vi "Radau5_Sim Time Check.vi"(8 "error in (no error)":errorcluster, 9 "Allow reverse?":bool, 10 "Final time":dbl, 11 "Initial time":dbl) -> (0 "error out":errorcluster)   [LabVIEW 2017, in "NI_DAE.lvlib"]
uses:
  <vilib>/gmath/NI_DAE.lvlib
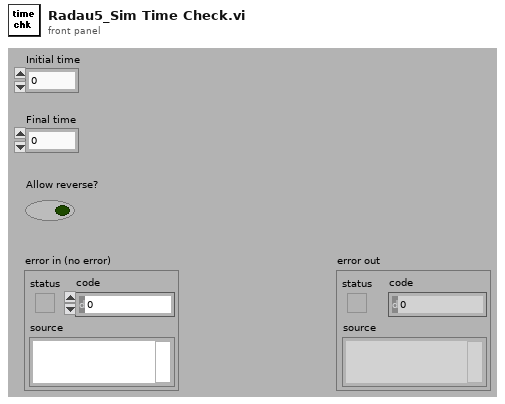
[diagram p1: front panel]
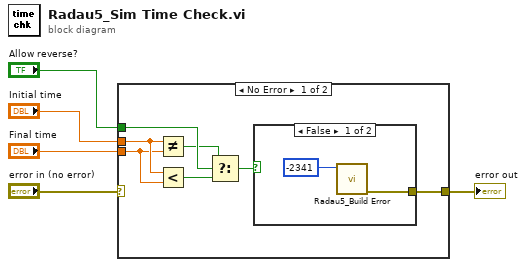
[diagram p0: block diagram]
diagram:
  n1 = case shown="No Error" "error in (no error)" {
    selector: "error in (no error)" -> [_ w15]
    tunnel: "Initial time" -> [w12 _]
    tunnel: "Final time" -> [w11 _]
    tunnel: "Allow reverse?" -> [w10 _]
    tunnel: [w6 w15] -> w1
    frame No Error {
      n2 = Not Equal?(x=w12, y=w11) -> (x != y?=w9:bool)
      n3 = Less?(x=w12, y=w11) -> (x < y?=w8:bool)
      n4 = Select(t=w9, s=w10, f=w8) -> (s? t:f=w7:bool)
      n5 = case shown="False" w7 {
        tunnel: [w13 _] -> w6
        frame False {
          n6 = call <vilib>:"Radau5_Build Error.vi"("error code"=-2341 ("error.code")) -> ("error out"=w13:errorcluster)  [unwired: 10 in]
        }
        frame True {
        }
      }
    }
    frame Error {
    }
  }
  "error out" <- w1
